vi "maxVelItCanAchieve.vi"(0 "Game in":refnum<class "Game.lvclass">, 5 "error in (no error)":errorcluster, 8 "distRobotNextDest":dbl format="%0.2f", 9 "robotModel":dbl[][](array[numeric]), 10 "est_vel":dbl[](array[numeric]), 12 "delta":dbl=0.2 format="%#_13g") -> (14 "Game out":refnum<class "Game.lvclass">, 16 "maxVelPossibleAtNextDest":dbl, 19 "error out":errorcluster)   [LabVIEW 2020, in "Game.lvclass"]
uses:
  Game.lvclass
  <vilib>/Analysis/_algsub.llb/Real Vector Norm.vi
  <vilib>/Analysis/NI_AALPro.lvlib
panel:
  in  "L":dbl format="%#_13g"
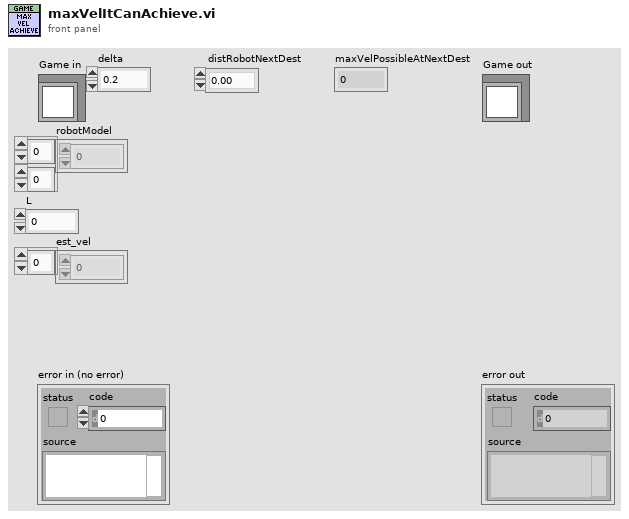
[diagram p1: front panel]
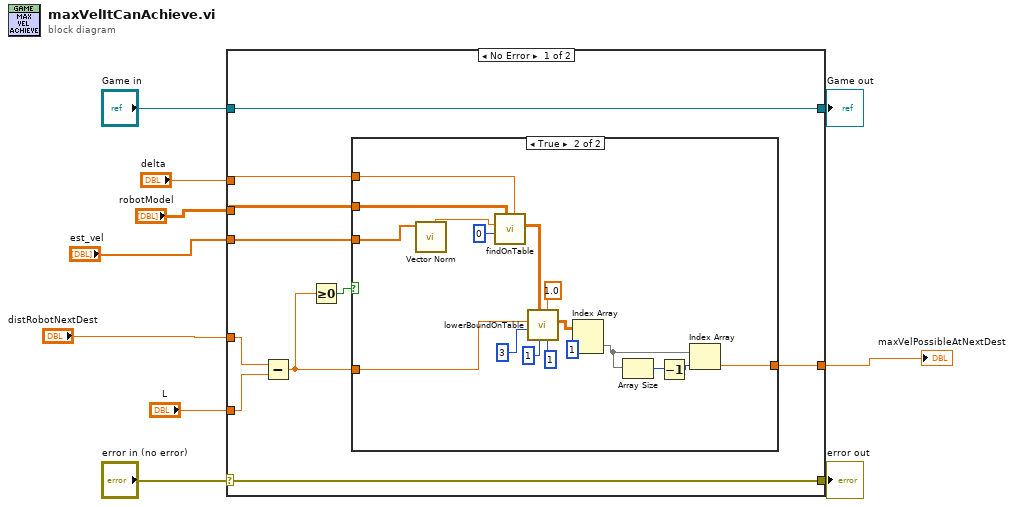
[diagram p0: block diagram]
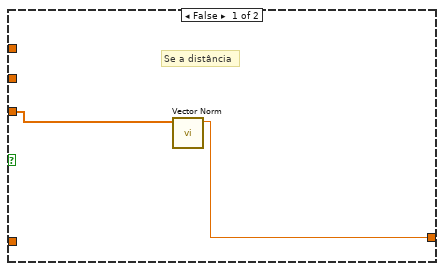
[diagram p2: hidden frame]
diagram:
  n1 = case shown="No Error" "error in (no error)" {
    selector: "error in (no error)" -> [w19 w41]
    tunnel: [w19 w41] -> w9
    tunnel: [w20 w40] -> w7
    tunnel: "Game in" -> [w20 w40]
    tunnel: "robotModel" -> [w15 _]
    tunnel: "L" -> [w17 _]
    tunnel: "distRobotNextDest" -> [w18 _]
    tunnel: "est_vel" -> [w16 _]
    tunnel: "delta" -> [w14 _]
    tunnel: [w13 _] -> w1
    frame No Error {
      n2 = Subtract(x=w18, y=w17) -> (x-y=w12:dbl)
      n3 = Greater Or Equal To 0?(x=w12) -> (x >= 0?=w11:bool)
      n4 = case shown="True" w11 {
        tunnel: w12 -> [_ w35]
        tunnel: w16 -> [w22 w31]
        tunnel: w15 -> [_ w29]
        tunnel: w14 -> [_ w28]
        tunnel: [w21 w24] -> w13
        frame False {
          # "Se a distância"
          n5 = call-poly <vilib>:"Vector Norm.vi"("Input Vector"=w22) -> ("norm"=w21:dbl)  [unwired: 9 in, 1 out]
        }
        frame True {
          n6 = call-poly <vilib>:"Vector Norm.vi"("Input Vector"=w31) -> ("norm"=w23:dbl)  [unwired: 9 in, 1 out]
          n7 = call "findOnTable.vi"("delta"=w28, "table"=w29, "column"=0, "key"=w23) -> ("search_results"=w27:dbl[][])  [unwired: 5 in, 2 out]
          n8 = call "lowerBoundOnTable.vi"("column_to_sort"=1, "sign"=1.0, "sign_idx"=1, "table"=w27, "target_idx"=3, "key"=w35) -> ("search_results"=w34:dbl[][])  [unwired: 3 in, 2 out]
          n9 = Index Array(array=w34, index (col)=1 ("disabled index (col)")) -> (element=w32:dbl[])  [unwired: 1 in]
          n10 = Array Size(array=w32) -> (size(s)=w26:i32)
          n11 = Decrement(x=w26) -> (x-1=w25:i32)
          n12 = Index Array(array=w32, index=w25) -> (element=w24:dbl)
        }
      }
    }
    frame Error {
    }
  }
  "error out" <- w9
  "Game out" <- w7
  "maxVelPossibleAtNextDest" <- w1
